vi "Destroy.vi"(0 "reference in":refnum<class "Executer.lvclass">, 5 "error in (no error)":errorcluster) -> (14 "reference out":refnum<class "Executer.lvclass">, 19 "error out":errorcluster)   [LabVIEW 2018, in "Executer.lvclass"]
uses:
  Executer.lvclass
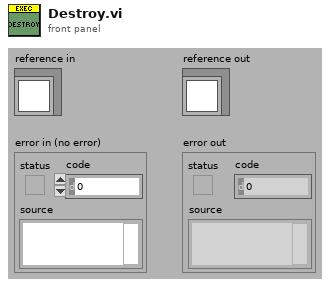
[diagram p1: front panel]
types:
  T1 = typedef "Executer.lvclass/ObjectAttributes.ctl" = cluster{"Executions":T2[]}
  T2 = typedef "Executer.lvclass/ClassExecutionInfo.ctl" = cluster{"Class":refnum<class>, "ClassName":string, "VIExecutionInfo":T3[]}
  T3 = typedef "Executer.lvclass/MethodExecutionInfo.ctl" = cluster{"viRef":refnum<vi>, "MethodName":string, "ControlIndices":i32[], "ClassInIndex":i32, "IndicatorIndices":i32[], "ErrorOutIndex":i32, "ControlTypes":variant[]}
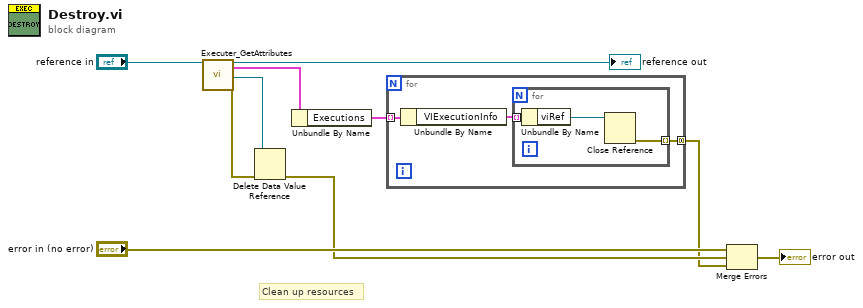
[diagram p0: block diagram]
diagram:
  # "Clean up resources"
  n1 = call "Executer_GetAttributes.vi"("reference in"="reference in") -> ("reference out"=→"reference out":refnum<class "Executer.lvclass">, "Data"=w5:T1, "DataRef"=w6:refnum<data-value>, "error out"=w7:errorcluster)  [unwired: 15 in]
  n2 = Delete Data Value Reference(data value reference=w6, error in=w7) -> (error out=w3:errorcluster)  [unwired: 1 out]
  n3 = Unbundle By Name(w5) -> ("Executions"=w2:T2[])
  n4 = for {
    tunnel: w2 -> [w13] mode=indexing
    tunnel: [w12] -> w1 mode=concatenating
    n5 = Unbundle By Name(w13) -> ("VIExecutionInfo"=w11:T3[])
    n6 = for {
      tunnel: w11 -> [w16] mode=indexing
      tunnel: [w15] -> w12 mode=indexing
      n7 = Unbundle By Name(w16) -> ("viRef"=w14:refnum<vi>)
      n8 = Close Reference(reference=w14) -> (error out=w15:errorcluster)  [unwired: 1 in]
    }
  }
  n9 = Merge Errors("error in (no error)", w3, w1) -> (→"error out":errorcluster)
